vi "Join Node and Link sections.vi"() -> (0 "string":string)   [LabVIEW 2018, in "DGML creation.lvlib"]
uses:
  DGML creation.lvlib
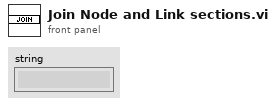
[diagram p1: front panel]
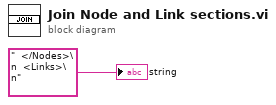
[diagram p0: block diagram]
diagram:
  "string" <- "  </Nodes>\n  <Links>\n" ("string")
